vi "Send client commands.vi"(8 "error in (no error)":errorcluster, 11 "Control-Client in":refnum<class "Control-Client.lvclass">) -> (0 "error out":errorcluster, 3 "Control-Client out":refnum<class "Control-Client.lvclass">)   [LabVIEW 2015, in "Control-Client.lvclass"]
uses:
  Control-Client.lvclass
  Control-Client.lvclass/Control-Client.ctl
  dependecies/ControlsVIs/Clusters-def/Message types.ctl
  dependecies/ControlsVIs/Clusters-def/Standard Command.ctl
  <vilib>/NI/STM/TCP/Write Message (TCP).vi
  <vilib>/NI/STM/NI STM.lvlib
  Message/Message.lvclass
  GeneralFunctionality/GeneralFunctionality.lvclass
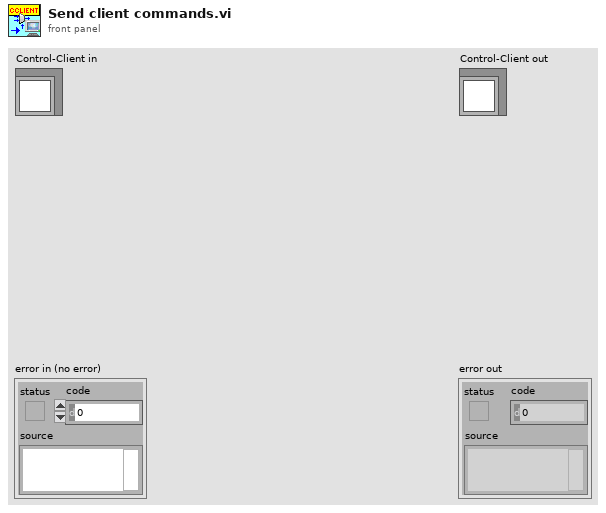
[diagram p1: front panel]
types:
  T1 = typedef "Message types.ctl" = string
  T2 = typedef "Standard Command.ctl" = cluster{"command":string, "data":variant}
  T3 = typedef "NI STM.lvlib/TCP Connection Info.ctl" = cluster{"connection ID":refnum<k5>, "meta data":T4[]}
  T4 = typedef "NI STM.lvlib/MetaDataElement.ctl" = string
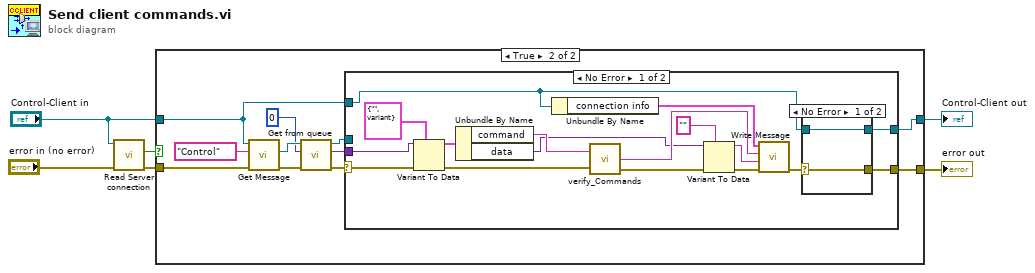
[diagram p0: block diagram]
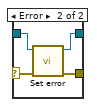
[diagram p3: hidden frame]
diagram:
  n1 = call "Read Server connection.vi"("error in (no error)"="error in (no error)", "Control-Client in"="Control-Client in") -> ("error out"=w2:errorcluster, "Server connection"=w3:bool)  [unwired: 7 in, 1 out]
  n2 = case shown="True" w3 {
    tunnel: [w8 w11] -> w5
    tunnel: "Control-Client in" -> [w7 w9]
    tunnel: w2 -> [w8 w16]
    tunnel: [w7 w10] -> w1
    frame False {
    }
    frame True {
      n3 = call "Get Message.vi"("error in (no error)"=w16, "Message type"=T1 "Control", "GeneralFunctionality en entrée"=w9) -> ("error out"=w19:errorcluster, "Message.lvclass"=w18:refnum<class "Message.lvclass">)  [unwired: 6 in, 1 out]
      n4 = call "Get from queue.vi"("error in (no error)"=w19, "timeout in ms (-1)"=0, "Message in"=w18) -> ("error out"=w14:errorcluster, "Data"=w17:variant, "Message out"=w13:refnum<class "Message.lvclass">)  [unwired: 6 in]
      n5 = case shown="No Error" w14 {
        selector: w14 -> [w35 w44]
        tunnel: w17 -> [w36 _]
        tunnel: [w31 w44] -> w11
        tunnel: w13 -> [_ _]
        tunnel: w9 -> [w29 w43]
        tunnel: [w30 w43] -> w10
        frame No Error {
          n6 = Variant To Data(error in=w35, type=T2 {"command"="", "data"=variant} ("input cluster"), Variant=w36) -> (data=w33:T2, error out=w27:errorcluster)
          n7 = Unbundle By Name(w33) -> ("command"=w28:string, "data"=w24:variant)
          n8 = Unbundle By Name(w29) -> ("connection info"=w34:T3)
          n9 = call "verify_Commands.vi"("Command"=w28, "error in"=w27) -> ("Command out"=w26:string, "error out"=w23:errorcluster)  [unwired: 1 out]
          n10 = Variant To Data(error in=w23, type="", Variant=w24) -> (data=w21:string, error out=w22:errorcluster)
          n11 = call-poly <vilib>:"Write Message.vi"("error in"=w22, "data"=w21, "name"=w26, "connection info in"=w34) -> ("error out"=w32:errorcluster)  [unwired: 6 in, 1 out]
          n12 = case shown="No Error" w32 {
            selector: w32 -> [w38 w40]
            tunnel: w29 -> [w37 w42]
            tunnel: [w38 w41] -> w31
            tunnel: [w37 w39] -> w30
            frame No Error {
            }
            frame Error {
              n13 = call "Set error.vi"("error in (no error)"=w40, "Control-Client in"=w42) -> ("error out"=w41:errorcluster, "Control-Client out"=w39:refnum<class "Control-Client.lvclass">)  [unwired: 8 in]
            }
          }
        }
        frame Error {
        }
      }
    }
  }
  "error out" <- w5
  "Control-Client out" <- w1
